vi "VisualizePodVectors_v2.vi"(10 "Pod Output Vectors":cluster{"Magnitude":dbl, "Direction":dbl}[](array[cluster]), 11 "Picture in":refnum<vi>) -> ()   [LabVIEW 2014]
uses:
  <vilib>/Analysis/coordinate.llb/3D Coordinate Conversion (Scalar).vi
  Variables/Physical data.vi
  <vilib>/Analysis/NI_AALPro.lvlib
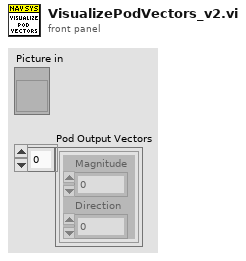
[diagram p1: front panel]
types:
  T1 = typedef "NI_Matrix.lvlib/RealMatrix.ctl" = dbl[][]
  T2 = cluster{"All Pod State Data":cluster{"Drive":cluster{"Drive Motor Output":dbl, "Wheel RPM":dbl, "Linear speed":dbl, "Linear acceleration":dbl, "Encoder Output":dbl, "Vmot":dbl, "Imot":dbl, "Torque":dbl, "Angular Momentum":dbl}, "Turret":cluster{"Turret Motor Output":dbl, "Turret Angle":dbl, "Turret velocity":dbl, "Turret acceleration":dbl, "Encoder Output":dbl, "Vmot":dbl, "Imot":dbl, "Torque":dbl, "Angular Momentum":dbl}, "Pod position (RCS)":cluster{"X":dbl, "Y":dbl, "Z":dbl}}[], "Global Robot Data":cluster{"Position Data":cluster{"Robot Position":cluster{"X":dbl, "Y":dbl, "Z":dbl}, "Robot Velocity":cluster{"X":dbl, "Y":dbl, "Z":dbl}, "Robot Acceleration":cluster{"X":dbl, "Y":dbl, "Z":dbl}}, "Rotation Data":cluster{"Angular Position":cluster{"X":dbl, "Y":dbl, "Z":dbl}, "Angular Velocity":cluster{"X":dbl, "Y":dbl, "Z":dbl}, "Angular Acceleration":cluster{"X":dbl, "Y":dbl, "Z":dbl}}}, "Inertial Characteristics":cluster{"Center of Mass (RCS)":cluster{"X":dbl, "Y":dbl, "Z":dbl}, "Mass Elements":cluster{"X":dbl, "Y":dbl, "Z":dbl, "Mass":dbl, "Name":string}[], "Center of Rotation (RCS)":cluster{"X":dbl, "Y":dbl, "Z":dbl}, "Tensor of Inertia":T1}}
  T3 = cluster{"PodConfigurations":cluster{"Drive":cluster{"Encoder":cluster{"CPft":dbl, "Location":string, "RIO_PinA":i32, "RIO_PinB":i32, "Invert?":bool}, "Motor":cluster{"PID":cluster{"P":dbl, "I":dbl, "D":dbl}, "CANorPWM Channel":i32, "Invert?":bool, "IsCanSRX?":bool, "Output":cluster{"Max":dbl, "Min":dbl}}}, "Turret":cluster{"Encoder":cluster{"ZeroPosVolts":dbl, "Location":string, "RIO_AnalogChannel":i32, "Invert?":bool}, "Motor":cluster{"PID":cluster{"P":dbl, "I":dbl, "D":dbl}, "CANorPWM Channel":i32, "Invert?":bool, "IsCanSRX?":bool, "Output":cluster{"Max":dbl, "Min":dbl}}}, "Misc":cluster{"Pod_Pos":cluster{"X":dbl, "Y":dbl}, "PDP_Channels":cluster{"Drive":i32, "Turret":i32}}}[], "General Configuration":cluster{"Pod Count":i32, "PDP CAN ID":i32, "PCM CAN ID":i32, "BaseRobotMass":dbl}}
  T4 = cluster{"Drive":cluster{"Encoder":cluster{"CPft":dbl, "Location":string, "RIO_PinA":i32, "RIO_PinB":i32, "Invert?":bool}, "Motor":cluster{"PID":cluster{"P":dbl, "I":dbl, "D":dbl}, "CANorPWM Channel":i32, "Invert?":bool, "IsCanSRX?":bool, "Output":cluster{"Max":dbl, "Min":dbl}}}, "Turret":cluster{"Encoder":cluster{"ZeroPosVolts":dbl, "Location":string, "RIO_AnalogChannel":i32, "Invert?":bool}, "Motor":cluster{"PID":cluster{"P":dbl, "I":dbl, "D":dbl}, "CANorPWM Channel":i32, "Invert?":bool, "IsCanSRX?":bool, "Output":cluster{"Max":dbl, "Min":dbl}}}, "Misc":cluster{"Pod_Pos":cluster{"X":dbl, "Y":dbl}, "PDP_Channels":cluster{"Drive":i32, "Turret":i32}}}[]
  T5 = cluster{"Coords":cluster{"X":dbl, "Y":dbl}, "Vector":cluster{"X":dbl, "Y":dbl}, "Hi-Speed?":bool}
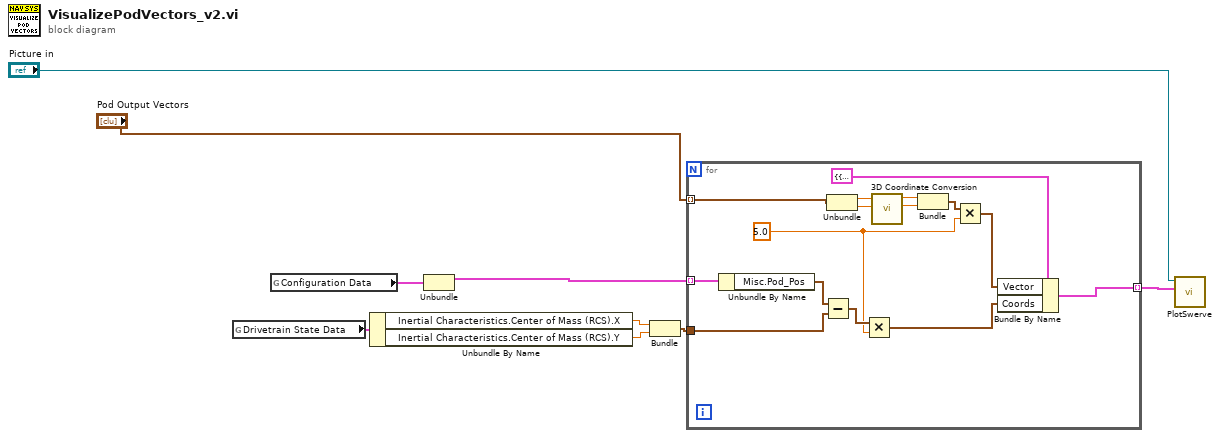
[diagram p0: block diagram]
diagram:
  n1 = global read "Physical data.vi" "Drivetrain State Data"() -> (w5:T2)
  n2 = global read "Physical data.vi" "Configuration Data"() -> (w3:T3)
  n3 = Unbundle By Name(w5) -> ("Inertial Characteristics.Center of Mass (RCS).X"=w7:dbl, "Inertial Characteristics.Center of Mass (RCS).Y"=w6:dbl)
  n4 = Unbundle(w3) -> ("PodConfigurations"=w4:T4)  [unwired: 1 out]
  n5 = Bundle("X"=w7, "Y"=w6) -> (w8:cluster{"X":dbl, "Y":dbl})  [unwired: 1 in]
  n6 = for {
    tunnel: "Pod Output Vectors" -> [w13] mode=indexing
    tunnel: [w23] -> w2 mode=indexing
    tunnel: w4 -> [w22] mode=indexing
    tunnel: w8 -> [w20]
    w10 = 5.0
    n7 = Unbundle By Name(w22) -> ("Misc.Pod_Pos"=w21:cluster{"X":dbl, "Y":dbl})
    n8 = Subtract(x=w21, y=w20) -> (x-y=w19:cluster{"X":dbl, "Y":dbl})
    n9 = Unbundle(w13) -> ("Magnitude"=w17:dbl, "Direction"=w16:dbl)
    n10 = Multiply(x=w19, y=w10) -> (x*y=w18:cluster{"X":dbl, "Y":dbl})
    n11 = call-poly <vilib>:"3D Coordinate Conversion.vi"("axis 2"=w16, "axis 1"=w17) -> ("axis 2 out"=w14:dbl, "axis 1 out"=w15:dbl)  [unwired: 6 in, 2 out]
    n12 = Bundle("axis 1 out"=w15, "axis 2 out"=w14) -> (w12:cluster{"axis 1 out":dbl, "axis 2 out":dbl})  [unwired: 1 in]
    n13 = Multiply(x=w12, y=w10) -> (x*y=w11:cluster{"axis 1 out":dbl, "axis 2 out":dbl})
    n14 = Bundle By Name(cluster=T5 {"Coords"={"X"=0.0, "Y"=0.0}, "Vector"={"X"=0.0, "Y"=0.0}, "Hi-Speed?"=FALSE}, "Vector"=w11, "Coords"=w18) -> (w23:T5)
  }
  n15 = call "PlotSwerve.vi"("Pod Plot Data In"=w2, "Picture refrence"="Picture in") -> ()  [unwired: 10 in]
